vi "Dis Mod Get IMAQ Ref.vi"(0 "Display Index":i32, 11 "Error In":errorcluster) -> (4 "IMAQ Ref":T1, 15 "Error Out":errorcluster)   [LabVIEW 2020]
uses:
  <vilib>/vision/Image Controls.llb/IMAQ Image.ctl
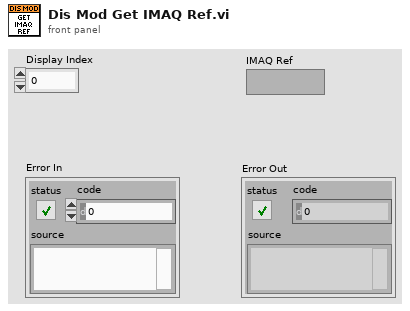
[diagram p1: front panel]
types:
  T1 = typedef "IMAQ Image.ctl" = refnum<image>
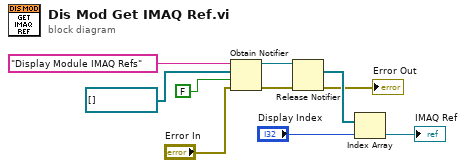
[diagram p0: block diagram]
diagram:
  n1 = Obtain Notifier(name (unnamed)="Display Module IMAQ Refs", notification data type=T1[] [], create if not found? (T)=FALSE, error in (no error)="Error In") -> (notifier out=w5:refnum<notifier>, error out=w4:errorcluster)  [unwired: 1 out]
  n2 = Release Notifier(notifier=w5, error in (no error)=w4) -> (last notification=w3:T1[], error out=→"Error Out":errorcluster)  [unwired: 1 in, 1 out]
  n3 = Index Array(array=w3, index="Display Index") -> (element=→"IMAQ Ref":T1)
